vi "fancy new vi.vi"(5 "control something":T1, 8 "b":dbl, 9 "a":dbl) -> (1 "c":dbl)   [LabVIEW 2018]
uses:
  fancy new type.ctl
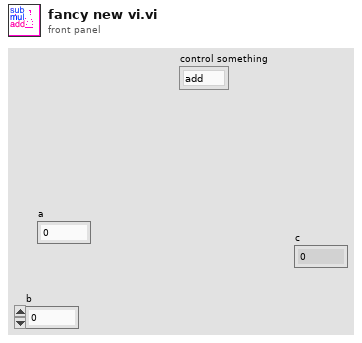
[diagram p1: front panel]
types:
  T1 = typedef "fancy new type.ctl" = enum16{"add", "sub", "mul"}
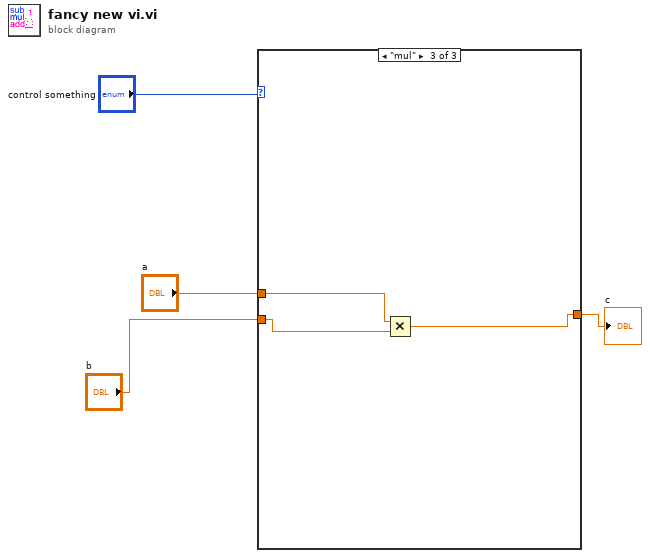
[diagram p0: block diagram]
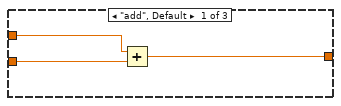
[diagram p2: hidden frame]
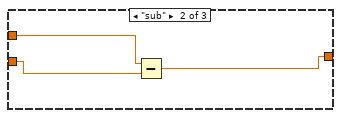
[diagram p3: hidden frame]
diagram:
  n1 = case shown="\"mul\"" "control something" {
    tunnel: "a" -> [w7 w10 w13]
    tunnel: "b" -> [w6 w9 w12]
    tunnel: [w5 w8 w11] -> w1
    frame "add", Default {
      n2 = Add(x=w7, y=w6) -> (x+y=w5:dbl)
    }
    frame "sub" {
      n3 = Subtract(x=w10, y=w9) -> (x-y=w8:dbl)
    }
    frame "mul" {
      n4 = Multiply(x=w13, y=w12) -> (x*y=w11:dbl)
    }
  }
  "c" <- w1
